vi "test get cluster field names.vi"() -> ()   [LabVIEW 2018, in "LV-Julia_ZMQ-Roundtrip_lib.lvlib"]
uses:
  <vilib>/Utility/Data Type/Type Definitions/Data Type.ctl
  LV-Julia_ZMQ-Roundtrip_lib.lvlib
  <vilib>/Utility/Data Type/NI_Data Type.lvlib
panel:
  out "Name 2":string
  out "Type 2":T1
  out "Name":string
  out "Type":T1
  out "Cluster Elements":variant[](array[variant])
  in  "error in (no error)":errorcluster
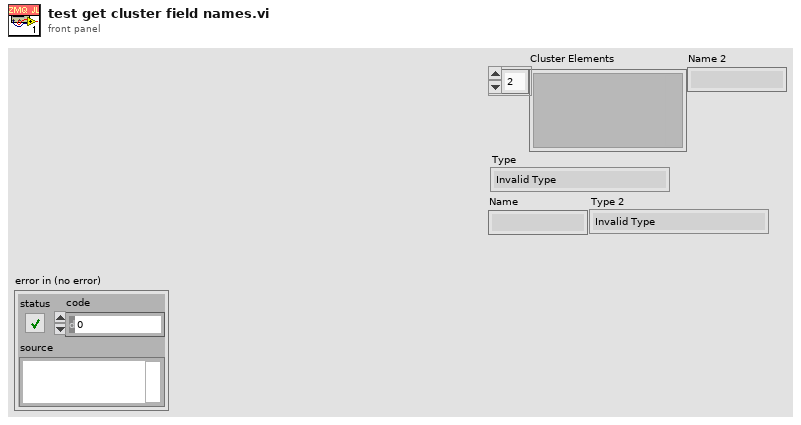
[diagram p1: front panel]
types:
  T1 = typedef "NI_Data Type.lvlib/Data Type.ctl" = enum8{"Invalid Type", "Void", "I8", "I16", "I32", "I64", "U8", "U16", "U32", "U64", "Single Float", "Double Float", "Extended Float", "Single Complex", "Double Complex", "Extended Complex", "Enum U8", "Enum U16", "Enum U32", "Enum U64", "Single Float With Unit", "Double Float With Unit", "Extended Float With Unit", "Single Complex with Unit", "Double Complex with Unit", "Extended Complex with Unit", "Boolean", "String", "Path", "Picture", "Tag", "Array", "Cluster", "Variant", "LV Variant", "Waveform", "Timestamp", "Digital Waveform", "Digital Data", "ExpressData", "Refnum", "External Data", "VI", "Poly VI", "LabVIEW Class Instance", "Fixed Point"}
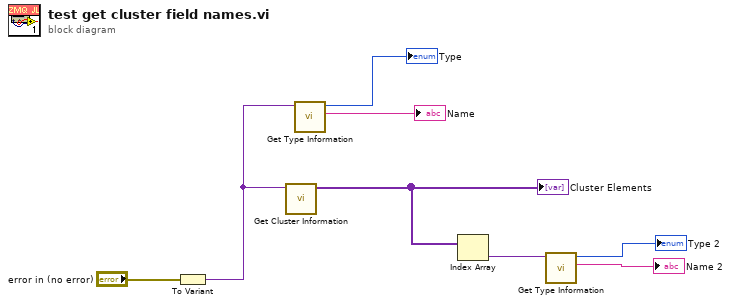
[diagram p0: block diagram]
diagram:
  n1 = To Variant(anything="error in (no error)") -> (Variant=w7:variant)
  n2 = call <vilib>:"Get Cluster Information.vi"("Variant"=w7) -> ("Cluster Elements"=w4:variant[])  [unwired: 9 in, 1 out]
  "Cluster Elements" <- w4
  n3 = call <vilib>:"Get Type Information.vi"("Variant"=w7) -> ("Name"=→"Name":string, "Type"=→"Type":T1)  [unwired: 6 in, 3 out]
  n4 = Index Array(array=w4) -> (element=w3:variant)  [unwired: 1 in]
  n5 = call <vilib>:"Get Type Information.vi"("Variant"=w3) -> ("Name"=→"Name 2":string, "Type"=→"Type 2":T1)  [unwired: 6 in, 3 out]
